vi "calculate_jsc.vi"(9 "wavelengths":dbl[](array[numeric]), 10 "eqe measurements":dbl[](array[numeric])) -> (2 "jsc (mA/cm^2)":dbl)   [LabVIEW 2018]
uses:
  <vilib>/Analysis/2dsp.llb/Integral Method.ctl
  <vilib>/Analysis/8numeric.llb/1D Numeric Integration.vi
  <vilib>/Utility/file.llb/Read Delimited Spreadsheet (DBL).vi
  <vilib>/gmath/NI_Gmath.lvlib
  <vilib>/Analysis/NI_AALPro.lvlib
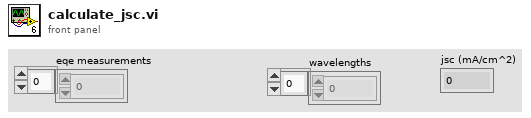
[diagram p1: front panel]
types:
  T1 = typedef "NI_AALPro.lvlib/Integral Method.ctl" = i32
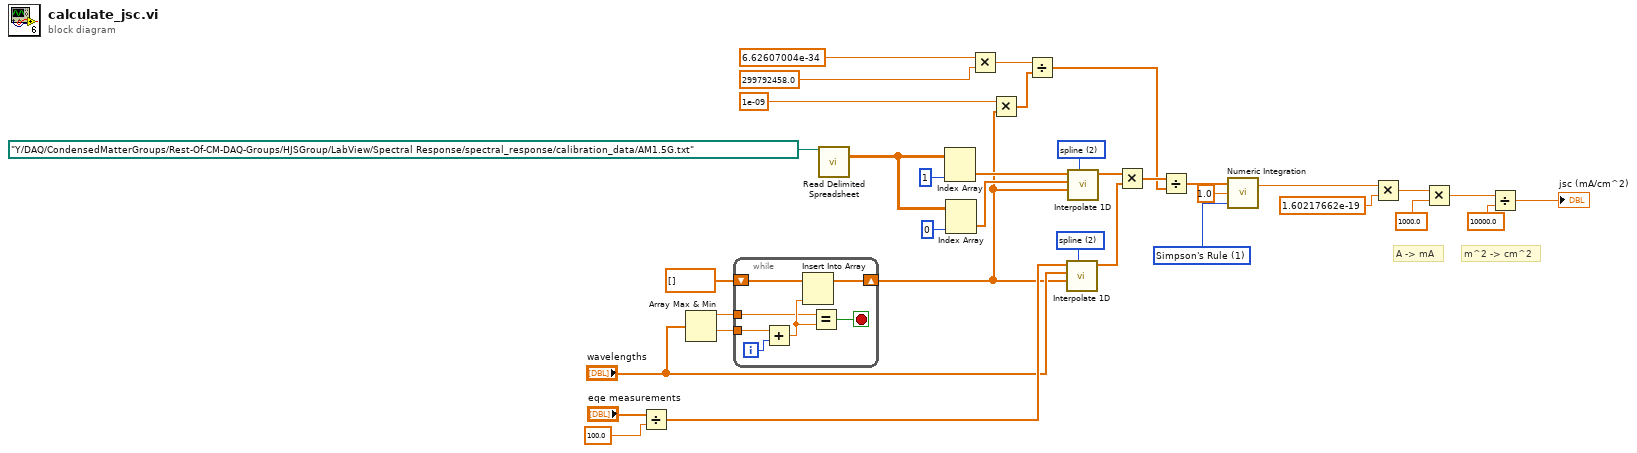
[diagram p0: block diagram]
diagram:
  w10 = 2 items=["nearest", "linear", "spline", "cubic Hermite", "Lagrange"] ("method")
  w16 = T1 1 items=["Trapezoidal Rule", "Simpson's Rule", "Simpson's 3/8 Rule", "Bode Rule"] ("integration method")
  w29 = 2 items=["nearest", "linear", "spline", "cubic Hermite", "Lagrange"] ("method")
  # "m^2 -> cm^2"
  # "A -> mA"
  n1 = Divide(x="eqe measurements", y=100.0) -> (x/y=w9:dbl[])
  n2 = Array Max & Min(array="wavelengths") -> (max value=w11:dbl, min value=w13:dbl)  [unwired: 2 out]
  n3 = while {
    tunnel: w13 -> [w41]
    shift-right: [w39] -> w7
    shift-left: dbl[] [] ("wavelengths") -> [w40]
    tunnel: w11 -> [w36]
    i -> [w42]
    stop <- w38 stop-if-true
    n4 = Add(x=w41, y=w42) -> (x+y=w37:dbl)
    n5 = Insert Into Array(array=w40, new element=w37) -> (w39:dbl[])  [unwired: 1 in]
    n6 = Equal?(x=w36, y=w37) -> (x = y?=w38:bool)
  }
  n7 = call-poly <vilib>:"Read Delimited Spreadsheet.vi"("file path (dialog if empty)"=path "Y:/DAQ/CondensedMatterGroups/Rest-Of-CM-DAQ-Groups/HJSGroup/LabView/Spectral Response/spectral_response/calibration_data/AM1.5G.txt" ("AM1.5G file path")) -> ("all rows"=w33:dbl[][])  [unwired: 9 in, 5 out]
  n8 = Index Array(array=w33, index (col)=1 ("disabled index (col)")) -> (element=w31:dbl[])  [unwired: 1 in]
  n9 = Index Array(array=w33, index (col)=0 ("index")) -> (element=w30:dbl[])  [unwired: 1 in]
  n10 = Multiply(x=6.62607004e-34, y=299792458.0) -> (x*y=w26:dbl)
  n11 = Multiply(x=1e-09 ("y"), y=w7) -> (x*y=w25:dbl[])
  n12 = Divide(x=w26, y=w25) -> (x/y=w19:dbl[])
  n13 = call <vilib>:"Interpolate 1D.vi"("method"=w10, "xi"=w7, "X"="wavelengths", "Y"=w9) -> ("yi"=w6:dbl[])  [unwired: 5 in, 2 out]
  n14 = call <vilib>:"Interpolate 1D.vi"("method"=w29, "xi"=w7, "X"=w30, "Y"=w31) -> ("yi"=w23:dbl[])  [unwired: 5 in, 2 out]
  n15 = Multiply(x=w23, y=w6) -> (x*y=w20:dbl[])
  n16 = Divide(x=w20, y=w19) -> (x/y=w17:dbl[])
  n17 = call-poly <vilib>:"Numeric Integration.vi"("integration method"=w16, "dt"=1.0, "Input Array"=w17) -> ("result"=w18:dbl)  [unwired: 1 out]
  n18 = Multiply(x=w18, y=1.60217662e-19) -> (x*y=w5:dbl)
  n19 = Multiply(x=w5, y=1000.0) -> (x*y=w3:dbl)
  n20 = Divide(x=w3, y=10000.0) -> (x/y=→"jsc (mA/cm^2)":dbl)
